vi "MTS_GenFileComment.vi"(5 "Parent File No":i32=-1, 6 "Time Per Pixel [ms]":dbl, 7 "Measurement Type":T2(ring)=enum."Image File", 8 "error in":errorcluster, 9 "Upper Left":T4, 10 "Pixels":i32[](array[numeric]), 11 "Picture Size":dbl[](array[numeric])) -> (0 "error out":errorcluster, 1 "Image Header":T1, 2 "Image Info":T3, 3 "Comment":string)   [LabVIEW 2010]
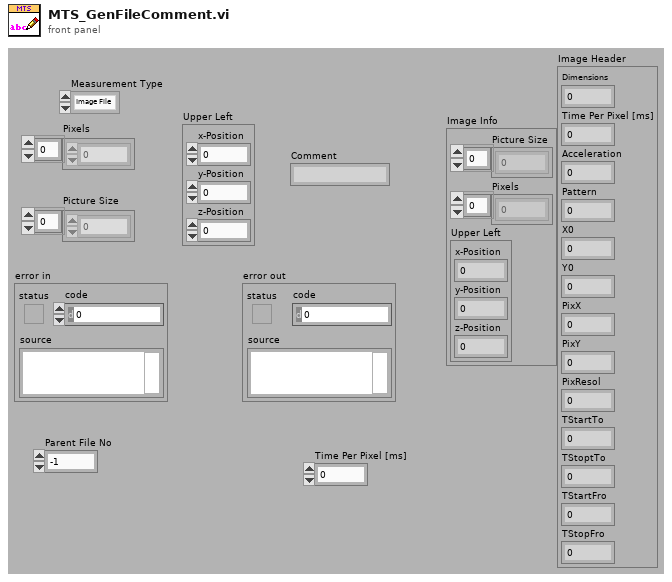
[diagram p1: front panel]
types:
  T1 = cluster{"Dimensions":i32, "Time Per Pixel [ms]":dbl, "Acceleration":i32, "Pattern":i32, "X0":sgl, "Y0":sgl, "PixX":i32, "PixY":i32, "PixResol":sgl, "TStartTo":sgl, "TStoptTo":sgl, "TStartFro":sgl, "TStopFro":sgl}
  T2 = enum16{"not a pt3 File", "Image File", "Point Measurement", "Auto Point", "Line Scan", "Grid Scan"}
  T3 = cluster{"Picture Size":dbl[], "Pixels":i32[], "Upper Left":cluster{"x-Position":dbl, "y-Position":dbl, "z-Position":dbl}}
  T4 = cluster{"x-Position":dbl, "y-Position":dbl, "z-Position":dbl}
  T5 = enum16{"not a pt3 File", "Image File", "Point Measurement", "Auto Point"}
  T6 = cluster{"File No":i32, "File Path":path, "Parent File":i32, "File Type":enum16{"unknown", "pt3 File", "png Image", "bmp Image"}, "Measurement Type":enum16{"not a pt3 File", "Image File", "Point Measurement", "Auto Point", "Line Scan", "Grid Scan"}, "Upper Left":cluster{"x-Position":dbl, "y-Position":dbl, "z-Position":dbl}, "Pixels":i32[], "Picture Size":dbl[], "Scan Axis":enum32{"x-y", "x-z", "y-z"}}
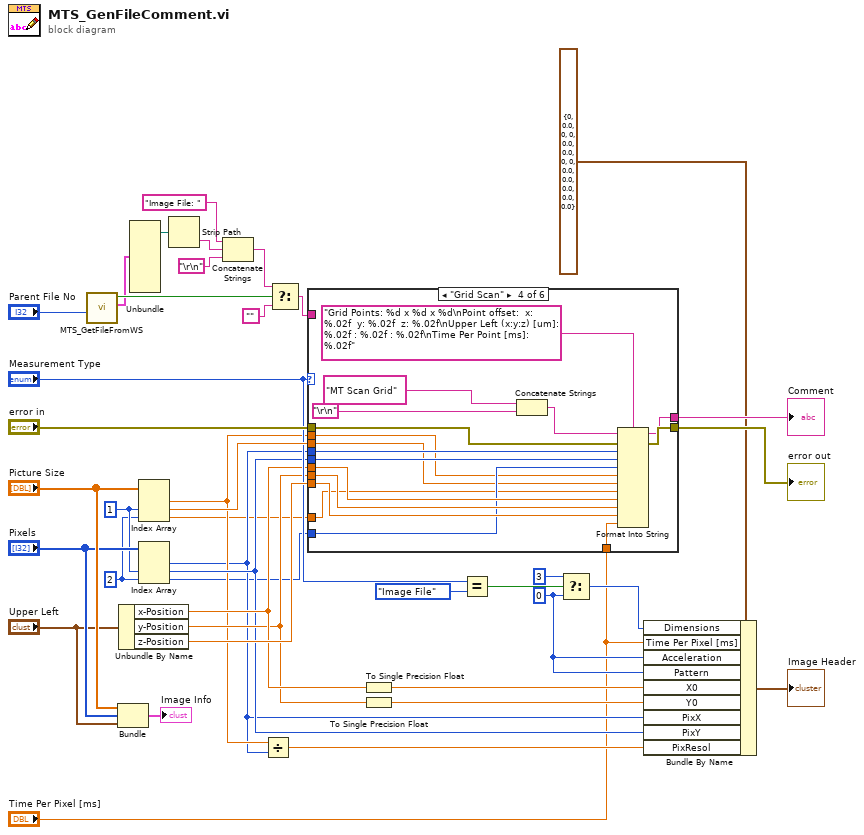
[diagram p0: block diagram]
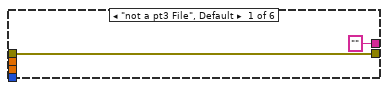
[diagram p2: hidden frame]
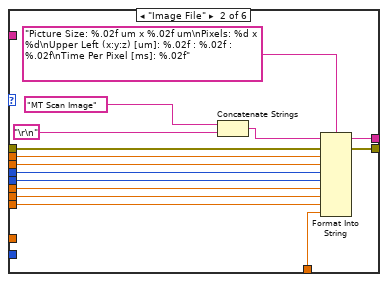
[diagram p3: hidden frame]
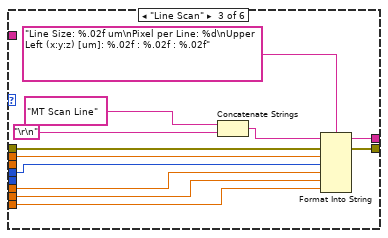
[diagram p4: hidden frame]
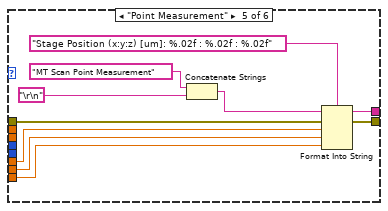
[diagram p5: hidden frame]
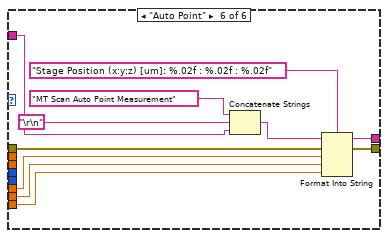
[diagram p6: hidden frame]
diagram:
  w24 = 0 ("f")
  w3 = 2 ("index")
  w4 = 1 ("index")
  n1 = call "MTS_GetFileFromWS.vi"("File No"="Parent File No") -> ("File Header"=w9:T6, "File Found"=w13:bool)  [unwired: 9 in]
  n2 = Bundle("Picture Size"="Picture Size", "Pixels"="Pixels", "Upper Left"="Upper Left") -> (→"Image Info":T3)  [unwired: 1 out]
  n3 = Unbundle By Name("Upper Left") -> ("x-Position"=w23:dbl, "y-Position"=w22:dbl, "z-Position"=w37:dbl)
  n4 = Unbundle(w9) -> ("File Path"=w8:path)  [unwired: 8 out]
  n5 = Index Array(array="Picture Size", index #2=w4, index #3=w3) -> (element #1=w18:dbl, element #2=w38:dbl, element #3=w2:dbl)  [unwired: 1 in]
  n6 = Index Array(array="Pixels", index #2=w4, index #3=w3) -> (element #1=w17:i32, element #2=w19:i32, element #3=w1:i32)  [unwired: 1 in]
  n7 = Strip Path(path=w8) -> (name=w6:string)  [unwired: 1 out]
  n8 = Concatenate Strings("Image File: " ("string"), w6, "\r\n") -> (w7:string)
  n9 = Divide(x=w18, y=w17) -> (x/y=w16:dbl)
  n10 = Select(t=w7, s=w13, f="") -> (s? t:f=w11:string)
  n11 = case shown="\"Grid Scan\"" "Measurement Type" {
    tunnel: [w42 w56 w68 w85 w95 w106] -> w40
    tunnel: "error in" -> [w42 w55 w67 w84 w94 w105]
    tunnel: w18 -> [_ w54 w66 w73 _ _]
    tunnel: w38 -> [_ w53 _ w71 _ _]
    tunnel: w17 -> [_ w52 w61 w76 _ _]
    tunnel: w19 -> [_ w51 _ w75 _ _]
    tunnel: w23 -> [_ w50 w60 w79 w92 w103]
    tunnel: w22 -> [_ w49 w59 w78 w91 w102]
    tunnel: w37 -> [_ w48 w58 w77 w90 w101]
    tunnel: ["" w47 w65 w83 w93 w104] -> w36
    tunnel: "Time Per Pixel [ms]" -> [_ w43 _ w70 _ _]
    tunnel: w11 -> [_ _ _ _ _ w97]
    tunnel: w2 -> [_ _ _ w72 _ _]
    tunnel: w1 -> [_ _ _ w74 _ _]
    frame "not a pt3 File", Default {
    }
    frame "Image File" {
      n12 = Concatenate Strings("MT Scan Image" ("initial string"), "\r\n") -> (w44:string)
      n13 = Format Into String(format string="Picture Size: %.02f um x %.02f um\nPixels: %d x %d\nUpper Left (x:y:z) [um]: %.02f : %.02f : %.02f\nTime Per Pixel [ms]: %.02f", initial string=w44, error in=w55, w54, w53, w52, w51, w50, w49, w48, w43) -> (resulting string=w47:string, error out=w56:errorcluster)
    }
    frame "Line Scan" {
      n14 = Concatenate Strings("MT Scan Line" ("initial string"), "\r\n") -> (w62:string)
      n15 = Format Into String(format string="Line Size: %.02f um\nPixel per Line: %d\nUpper Left (x:y:z) [um]: %.02f : %.02f : %.02f", initial string=w62, error in=w67, w66, w61, w60, w59, w58) -> (resulting string=w65:string, error out=w68:errorcluster)
    }
    frame "Grid Scan" {
      n16 = Concatenate Strings("MT Scan Grid" ("initial string"), "\r\n") -> (w80:string)
      n17 = Format Into String(format string="Grid Points: %d x %d x %d\nPoint offset:  x: %.02f  y: %.02f  z: %.02f\nUpper Left (x:y:z) [um]: %.02f : %.02f : %.02f\nTime Per Point [ms]: %.02f", initial string=w80, error in=w84, w76, w75, w74, w73, w71, w72, w79, w78, w77, w70) -> (resulting string=w83:string, error out=w85:errorcluster)
    }
    frame "Point Measurement" {
      n18 = Concatenate Strings("MT Scan Point Measurement" ("initial string"), "\r\n") -> (w87:string)
      n19 = Format Into String(format string="Stage Position (x:y:z) [um]: %.02f : %.02f : %.02f", initial string=w87, error in=w94, w92, w91, w90) -> (resulting string=w93:string, error out=w95:errorcluster)
    }
    frame "Auto Point" {
      n20 = Concatenate Strings("MT Scan Auto Point Measurement" ("initial string"), "\r\n", w97) -> (w98:string)
      n21 = Format Into String(format string="Stage Position (x:y:z) [um]: %.02f : %.02f : %.02f", initial string=w98, error in=w105, w103, w102, w101) -> (resulting string=w104:string, error out=w106:errorcluster)
    }
  }
  "error out" <- w40
  "Comment" <- w36
  n22 = To Single Precision Float(number=w23) -> (single precision float=w21:sgl)
  n23 = To Single Precision Float(number=w22) -> (single precision float=w20:sgl)
  n24 = Equal?(x="Measurement Type", y=T5."Image File") -> (x = y?=w27:bool)
  n25 = Select(t=3, s=w27, f=w24) -> (s? t:f=w25:i32)
  n26 = Bundle By Name(cluster=T1 {"Dimensions"=0, "Time Per Pixel [ms]"=0.0, "Acceleration"=0, "Pattern"=0, "X0"=0.0, "Y0"=0.0, "PixX"=0, "PixY"=0, "PixResol"=0.0, "TStartTo"=0.0, "TStoptTo"=0.0, "TStartFro"=0.0, "TStopFro"=0.0} ("Image Header"), "Dimensions"=w25, "Time Per Pixel [ms]"="Time Per Pixel [ms]", "Acceleration"=w24, "Pattern"=w24, "X0"=w21, "Y0"=w20, "PixX"=w17, "PixY"=w19, "PixResol"=w16) -> (→"Image Header":T1)
